vi "Unbundle Code Cluster.vi"(11 "code chunks cluster":T1[](array[typedef])) -> (0 "temp":string[](array[string]), 1 "C code":string[](array[string]), 2 "Defines":string[](array[string]), 3 "Includes":string[](array[string]))   [LabVIEW 2014]
doc: "Flatten of all items each array together, it tooks array of clusters and concatenate each array, so we can start remove duplicates in includes or definitions, doesn't matter. Justo for simplyfication.\n\nExtract each cluster item as separate array, that whole function of this VI.\n- defines 1D array\n- incliudes 1D array\n- C code 1D array"
uses:
  types/LabVIEW Universal Transcriptor Cluster.ctl
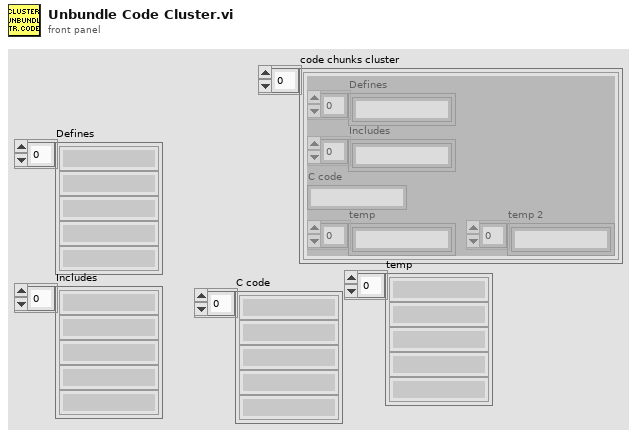
[diagram p1: front panel]
types:
  T1 = typedef "LabVIEW Universal Transcriptor Cluster.ctl" = cluster{"Defines":string[], "Includes":string[], "C code":string, "temp":string[], "temp 2":string[]}
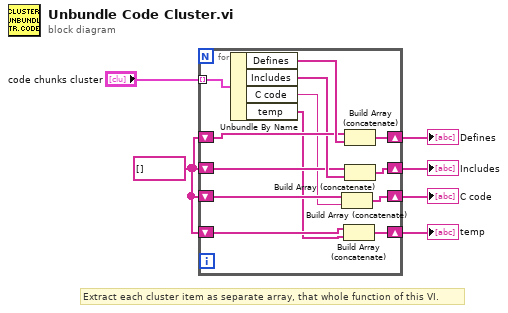
[diagram p0: block diagram]
diagram:
  w2 = string[] [] ("Defines")
  # "Extract each cluster item as separate array, that whole function of this VI."
  n1 = for {
    tunnel: "code chunks cluster" -> [w19] mode=indexing
    shift-right: [w17] -> w5
    shift-left: w2 -> [w16]
    shift-right: [w13] -> w4
    shift-left: w2 -> [w14]
    shift-right: [w10] -> w3
    shift-left: w2 -> [w12]
    shift-right: [w9] -> w1
    shift-left: w2 -> [w8]
    n2 = Unbundle By Name(w19) -> ("Defines"=w18:string[], "Includes"=w15:string[], "C code"=w11:string, "temp"=w7:string[])
    n3 = Build Array (concatenate)(w12, w11) -> (w10:string[])
    n4 = Build Array (concatenate)(w8, w7) -> (w9:string[])
    n5 = Build Array (concatenate)(w16, w18) -> (w17:string[])
    n6 = Build Array (concatenate)(w14, w15) -> (w13:string[])
  }
  "Defines" <- w5
  "Includes" <- w4
  "C code" <- w3
  "temp" <- w1
